vi "Protocol.Main.vi"(10 "Parameters":variant, 11 "Process":refnum<class "Process.lvclass">) -> ()   [LabVIEW 2023, in "J1939 Addon Engine.lvlib"]
uses:
  J1939 Addon Engine.lvlib
  <vilib>/NI/NIVS Inline Async API/_VS Inline Async API/Process/Process.lvclass
  Types/Protocol.App Settings.ctl
  Addon Shared/Types/XNET Settings.ctl
  Addon Shared/Types/Monitor Settings.ctl
  Types/Protocol.XNET Refs.ctl
  <vilib>/NI VeriStand/Custom Device API/Block Data Reference.ctl
  <vilib>/NI VeriStand/Custom Device API/Data Reference.ctl
  Types/Main.Outgoing.Frame.Settings.ctl
  Addon Shared/Types/Outgoing Event Trigger Types.ctl
  SubModules/Frame-Protection-Support/Source/Shared/Types/Exported Frame Settings.ctl
  SubModules/Frame-Protection-Support/Source/Shared/Types/Exported Frame Type.ctl
  SubModules/Frame-Protection-Support/Source/Shared/Types/Exported Protection Settings.ctl
  SubModules/Frame-Protection-Support/Source/Shared/Types/Protection Type.ctl
  SubModules/Frame-Protection-Support/Source/Shared/Types/XNET Signal Configuration.ctl
  SubModules/Frame-Protection-Support/Source/Shared/Types/Exported Counter Settings.ctl
  SubModules/Frame-Protection-Support/Source/Shared/Types/Exported Event Trigger Type.ctl
  Types/Engine.DTC Settings.ctl
  Addon Shared/Types/Compiled Simulated Settings.ctl
  Types/Engine.DTC FIFOs.ctl
  <vilib>/NI/NIVS Inline Async API/_VS Inline Async API/Process/Process.lvclass/Process.ctl
  <vilib>/NI/NI VeriStand Addon Network Comm/Engine/VeriStand Comm.lvclass/VeriStand Comm.ctl
  SubVIs/Protocol.Process Incoming Messages.vi
  <vilib>/NI/NIVS Inline Async API/_VS Inline Async API/Process/Methods/Async.Processes.Report.vi
  <vilib>/NI/NI VeriStand Addon Network Comm/Engine/_SubVIs/Comm Connection Engine.vi
  <vilib>/NI/NI VeriStand Addon Network Comm/Engine/_SubVIs/Comm Command Engine.vi
  SubVIs/Protocol.Process J1939 Incoming Messages.vi
  SubVIs/Protocol.RQST Lookup Table Act.vi
  <vilib>/NI/NI VeriStand Addon Network Comm/Engine/Comm API/Read Command.vi
  SubVIs/Protocol.RQST Wait on Response.vi
  SubVIs/Protocol.RQST Wait on Multiple Requests.vi
  Support Libraries/J1939 Utilities/Common Conversions.vi
  Support Libraries/J1939 Utilities/SubVIs/Convert CAN Arb ID to J1939 ID.vi
  SubModules/CAN-Streaming-Support/Source/Addon/Addon Engine/SubVIs/Reset Engine Stream Filter.vi
  SubModules/CAN-Streaming-Support/Source/Addon/Addon Engine/SubVIs/Get Engine Stream Filter.vi
  SubModules/CAN-Streaming-Support/Source/Addon/Addon Engine/SubVIs/Set Engine Stream Filter.vi
  SubVIs/Format Debug String.vi
  SubVIs/Protocol.Address Lookup Table Action.vi
  <vilib>/NI/NI VeriStand Addon Network Comm/Engine/Comm API/Respond to Command.vi
  <vilib>/Utility/error.llb/Clear Errors.vi
  SubModules/CAN-Streaming-Support/Source/Addon/Addon Engine/SubVIs/Engine Steam Format Debug String.vi
  SubModules/CAN-Streaming-Support/Source/Addon/Addon Engine/SubVIs/CAN Frame Filter.vi
  SubVIs/Protocol.Filter by Device Address.vi
  SubVIs/Protocol.Process Incoming Messages by PDU F.vi
  <vilib>/NI/NIVS Inline Async API/_VS Inline Async API/Error Handling Process/SubVIs/Error.ConvertArray.vi
  <vilib>/NI/STM/Connection Manager/TCP/Advanced/TCP Connection Manager (By Reference).vi
  <vilib>/NI/STM/Get Connection Reference.vi
  <vilib>/NI/STM/TCP/Get Connection Reference (TCP).vi
  <vilib>/NI/STM/Read Meta Data.vi
  <vilib>/NI/STM/TCP/Read Meta Data (TCP Ref).vi
  <vilib>/NI/AMC/Send Local Message.vi
  <vilib>/NI/Tools/Keyed Array/Add.vi
  <vilib>/NI/AMC/Read Next Message.vi
  <vilib>/NI/STM/Connection Manager/TCP/Advanced/TCP Check Connection (By Reference).vi
  SubVIs/Protocol.J1939 Filter by Device Address.vi
  <vilib>/NI/Tools/Keyed Array/Index.vi
  Support Libraries/J1939 Utilities/Common Messages.vi
  Support Libraries/J1939 Utilities/SubVIs/Request.vi
  SubVIs/Protocol.Parse Message Type.vi
  SubVIs/Protocol.RQST Look for Response.vi
  Support Libraries/J1939 Utilities/SubVIs/Convert J1939 ID to CAN Arb ID.vi
  Support Libraries/J1939 Utilities/SubVIs/Convert CAN Data (U32) to U8.vi
  SubVIs/Protocol.Get Simulated Previously Active DTCs.vi
  SubVIs/Protocol.Get Simulated Active DTCs.vi
  Support Libraries/J1939 Utilities/SubVIs/Acknowledgement.vi
  SubVIs/Protocol.Send Reset Previously Active DTC to Main.vi
  SubVIs/Protocol.Send Reset Active DTC to Main.vi
  SubVIs/Protocol.Convert Signals to Frame by ID.vi
  <vilib>/NI/STM/SubVIs/Generate STM Error.vi
  <vilib>/NI/AMC/Create Single Message.vi
  <vilib>/NI/AMC/Update Message Routing Info.vi
  <vilib>/NI/Tools/Keyed Array/Map String.vi
  <vilib>/NI/AMC/Read Termination Message.vi
  SubVIs/Protocol.Convert Data to DTC Frame.vi
  <vilib>/NI/Tools/String/Get Case Matching.vi
  <vilib>/xnet/xnet.llb/XNET Create Session.vi
  <vilib>/xnet/xnet.llb/XNET Create Session (Frame Input Stream).vi
  <vilib>/Utility/SystemLogging/Write to System Log.vi
  <vilib>/xnet/xnet.llb/XNET Read.vi
  <vilib>/xnet/xnet.llb/XNET Read (Frame CAN).vi
  <vilib>/xnet/xnet.llb/XNET Read (State CAN Comm).vi
  <vilib>/xnet/xnet.llb/XNET Clear.vi
  <vilib>/NI/NI VeriStand Addon Network Comm/Shared/Comm Constants.vi
  <vilib>/NI/AMC/Globals.vi
  <vilib>/Utility/error.llb/Error Cluster From Error Code.vi
  SubVIs/Protocol.RQST Lookup Table.vi
  SubVIs/Protocol.Address Lookup Table.vi
  <vilib>/NI/AMC/Send Message.vi
  <vilib>/xnet/xnet.llb/XNET Create Session (Conversion).vi
  <vilib>/xnet/xnet.llb/XNET Convert.vi
  <vilib>/xnet/xnet.llb/XNET Convert (Signal to Frame CAN).vi
  <vilib>/NI/STM/Read Message.vi
  <vilib>/NI/STM/TCP/Read Message (TCP).vi
  <vilib>/NI/AMC/Create Message Queue.vi
  <vilib>/NI/STM/Write Message.vi
  <vilib>/NI/STM/TCP/Write Message (TCP).vi
  <vilib>/NI/AMC/Destroy Message Queue.vi
  <vilib>/NI/STM/TCP/Read Meta Data (TCP Clst).vi
  SubVIs/Protocol.Close References.vi
  <vilib>/NI/NI VeriStand Addon Network Comm/Engine/Process/Close Comm Refs.vi
  <vilib>/NI/NI VeriStand Addon Network Comm/Engine/VeriStand Comm.lvclass
  Addon Shared/J1939 Addon Shared.lvlib
  <vilib>/NI VeriStand/Custom Device API/Custom Device API.lvlib
  SubModules/Frame-Protection-Support/Source/Shared/Protection and Counter Support Shared.lvlib
  SubModules/CAN-Streaming-Support/Source/Addon/Addon Engine/CAN Stream Support Engine.lvlib
panel:
  out "error out":errorcluster
  # "CONTROL & MONITORING"
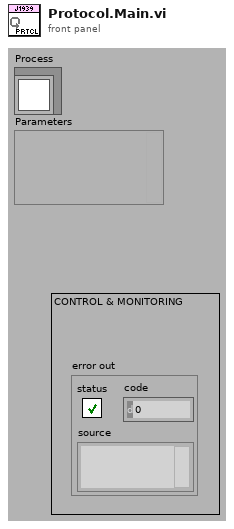
[diagram p1: front panel]
types:
  T1 = typedef "J1939 Addon Engine.lvlib/Protocol.App Settings.ctl" = cluster{"Name":string, "XNET.Settings":T2, "Monitor.Network":T3, "Data":T4[], "DTCs":T16[], "Sim.Nodes.LUT":variant, "Data.LUT":variant, "PCL":u32}
  T2 = typedef "J1939 Addon Shared.lvlib/XNET Settings.ctl" = cluster{"Database":refnum<k21>, "Cluster":refnum<k21>, "Port":string, "Baud rate [Bd]":u32, "Termination":u32, "Incoming Decimation":u32, "Outgoing Decimation":u32}
  T3 = typedef "J1939 Addon Shared.lvlib/Monitor Settings.ctl" = cluster{"Address":u8, "Name":u64, "Include DA":bool, "Force SA":bool}
  T4 = typedef "J1939 Addon Engine.lvlib/Protocol.XNET Refs.ctl" = cluster{"Network":T3, "Incoming.Use":bool, "Incoming.Session":refnum<k21>, "Incoming.Refs":T5[], "Incoming.Values":dbl[], "Outgoing.Frames":T7[], "Outgoing.Initialize":bool, "Outgoing.Refs":T5[], "Outgoing.Values":dbl[], "Request.Table":refnum<k33>, "Timing.Use":bool, "Timing.Index":i32[], "Timing.Refs":T5[], "Timing.Values":dbl[], "Disable.Refs":T5[], "Disable.Values":dbl[], "Trigger.Refs":T5[], "Trigger.Values":dbl[], "Outgoing.Frames.CountersAndProtections":T9[]}
  T5 = typedef "Custom Device API.lvlib/Block Data Reference.ctl" = cluster{"Data Reference":T6, "Offset":u64, "Length":u64}
  T6 = typedef "Custom Device API.lvlib/Data Reference.ctl" = i32
  T7 = typedef "J1939 Addon Engine.lvlib/Main.Outgoing.Frame.Settings.ctl" = cluster{"Offset":u32, "Length":u32, "Cyclic":bool, "Disable.Index":i32, "Disable":bool, "Trigger":T8, "Trigger.Index":i32, "Session":refnum<k21>}
  T8 = typedef "J1939 Addon Shared.lvlib/Outgoing Event Trigger Types.ctl" = enum16{"Channel value change", "Trigger channel (not zero)", "Channel value change or trigger channel (not zero)", "Trigger channel (any value change)", "Channel value change or trigger channel (any value change)"}
  T9 = typedef "Protection and Counter Support Shared.lvlib/Exported Frame Settings.ctl" = cluster{"Type":T10, "Frame ID":u32, "Payload Length":u32, "Signal XNET Paths":string[], "Frame.PrevData":dbl[], "VS Offset":i32, "VS Length":i32, "Generation Period":u32, "Has Protection?":bool, "Protection Configurations":T11[], "Has Counter":bool, "Counter Configurations":T14[], "Has Disable?":bool, "Disable VS Index":i32, "Transmit Trigger":T15, "Trigger VS Index":i32}
  T10 = typedef "Protection and Counter Support Shared.lvlib/Exported Frame Type.ctl" = enum16{"Periodic", "Event", "Periodic/Event"}
  T11 = typedef "Protection and Counter Support Shared.lvlib/Exported Protection Settings.ctl" = cluster{"Protection Frame Index":i32, "Protection Type":T12, "Data Indeces":i32[], "Initialized Data Array":dbl[], "Protection Signal XNET Paths":string[], "CRC Channels":T13[], "Protection VS Update Index":i32, "Override Index":i32, "Override Value Index":i32}
  T12 = typedef "Protection and Counter Support Shared.lvlib/Protection Type.ctl" = enum16{"Arb ID + Bytes Checksum with Inversion", "Arb ID + Bytes CRC with Inversion", "Reversed Raw Signal Checksum with Inversion", "Concatenated Two's Compliment"}
  T13 = typedef "Protection and Counter Support Shared.lvlib/XNET Signal Configuration.ctl" = cluster{"Start Bit":i32, "Name":string, "Number of bits":i32, "Scale":dbl, "Offset":dbl, "Data Type":u32, "Counter":bool}
  T14 = typedef "Protection and Counter Support Shared.lvlib/Exported Counter Settings.ctl" = cluster{"Frame Index":i32, "Max Count":dbl, "VS Index":i32, "Bit Length":i64, "Override Index":i32, "Override Value Index":i32}
  T15 = typedef "Protection and Counter Support Shared.lvlib/Exported Event Trigger Type.ctl" = enum16{"Channel value change", "Trigger channel (not zero)", "Channel value change or trigger channel (not zero)", "Trigger channel (any value change)", "Channel value change or trigger channel (any value change)"}
  T16 = typedef "J1939 Addon Engine.lvlib/Engine.DTC Settings.ctl" = cluster{"Data":T17, "FIFOs":T18}
  T17 = typedef "J1939 Addon Shared.lvlib/Compiled Simulated Settings.ctl" = cluster{"DM1.Ref":T5[], "DM1.Value":dbl[], "DM1.Enable.Ref":T5[], "DM1.Enable.Value":dbl[], "DM2.Ref":T5[], "DM2.Value":dbl[], "DM2.Enable.Ref":T5[], "DM2.Enable.Value":dbl[]}
  T18 = typedef "J1939 Addon Engine.lvlib/Engine.DTC FIFOs.ctl" = cluster{"DM1.Data":refnum<k33>, "DM1.Enable":refnum<k33>, "DM2.Data":refnum<k33>, "DM2.Enable":refnum<k33>, "DM1.Reset":refnum<k33>, "DM2.Reset":refnum<k33>}
  T19 = typedef "J1939 Addon Engine.lvlib/Protocol.Configuration.ctl" = cluster{"Refs":T20, "XNET":T23, "Comm":refnum<class "VeriStand Comm.lvclass">, "Process":refnum<class "Process.lvclass">, "Name":string, "InternalCmd":T24, "InternalResp":T25, "Resp.Data":dbl[], "CounterProtection":T26[], "Stream Refs":T29}
  T20 = typedef "J1939 Addon Engine.lvlib/Protocol.Refs.ctl" = cluster{"Processed Outgoing":refnum<queue>, "Simulated Addresses LUT":variant, "Data LUT":variant, "RequestDataTables":refnum<k33>[], "RQST":T21, "Address LUT":T22, "Addresses":u8[], "Monitor Address":u8}
  T21 = typedef "J1939 Addon Engine.lvlib/Protocol.RQST Lookup Table Reference.ctl" = refnum<data-value>
  T22 = typedef "J1939 Addon Engine.lvlib/Protocol.Address Table Reference.ctl" = refnum<data-value>
  T23 = typedef "J1939 Addon Engine.lvlib/Protocol.XNET Settings.ctl" = cluster{"Raw CAN In":refnum<k21>, "Raw Frames out":refnum<k21>[], "Raw J1939 In":refnum<k21>}
  T24 = typedef "Data Access Engine.lvlib/Data Access Engine.lvclass/Read.DVR.ctl" = refnum<data-value>
  T25 = typedef "Data Access Engine.lvlib/Data Access Engine.lvclass/Write.DVR.ctl" = refnum<data-value>
  T26 = typedef "J1939 Addon Engine.lvlib/CounterAndProtectionFrames.ctl" = cluster{"Frame Count":i32, "Frames in":T27[], "Protections":T25, "Signals":T24, "Overrides":T24}
  T27 = typedef "Protection and Counter Support Engine.lvlib/RT Frame Settings.ctl" = cluster{"Type":T10, "Frame ID":u32, "Payload Length":u32, "VS Offset":i32, "VS Length":i32, "Frame Conversion":refnum<k21>, "Frame.Data":dbl[], "Generation Period":u32, "Time Since Last Generation":u32, "Generation Iterations":u32, "Generation Counter":u32, "Has Protection?":bool, "Protection Configurations":T28[], "Has Counter?":bool, "Counter Configurations":T14[], "Has Disable?":bool, "Disable VS Index":i32, "Transmit Trigger":T15, "Trigger VS Index":i32}
  T28 = typedef "Protection and Counter Support Engine.lvlib/RT Protection Configuration.ctl" = cluster{"Protection Frame Index":i32, "Protection Type":T12, "Data Indeces":i32[], "Data Array":dbl[], "Check Sum Conversion":refnum<k21>, "CRC Channels":T13[], "Protection VS Index":i32, "Counter Data Index":i32, "Override Index":i32, "Override Value Index":i32}
  T29 = typedef "CAN Stream Support Engine.lvlib/Engine Stream Refs.ctl" = cluster{"Addon":string, "Port":refnum<k21>, "Filter Ref":refnum<data-value>, "Default Filter":T30, "Port Settings":T33}
  T30 = typedef "CAN Stream Support Shared.lvlib/Filter Parameters.ctl" = cluster{"ID Filters":u32[], "Direction Filter":T31, "Type Filter":T32}
  T31 = typedef "CAN Stream Support Shared.lvlib/Direction Filter.ctl" = enum16{"Tx/Rx", "Rx", "Tx"}
  T32 = typedef "CAN Stream Support Shared.lvlib/Type Filter.ctl" = enum16{"All", "CAN Data", "CAN Remote", "CAN Bus Error", "CAN 2.0 Data", "CAN FD Data", "CAN FD+BRS Data", "J1939 Data", "Delay", "Log Trigger", "Start Trigger"}
  T33 = typedef "CAN Stream Support Engine.lvlib/Engine Stream Port Settings.ctl" = cluster{"Mode":u32, "Baud Rate":u64, "Termination":u32, "FD ISO Mode":u32, "FD Baud Rate":u64}
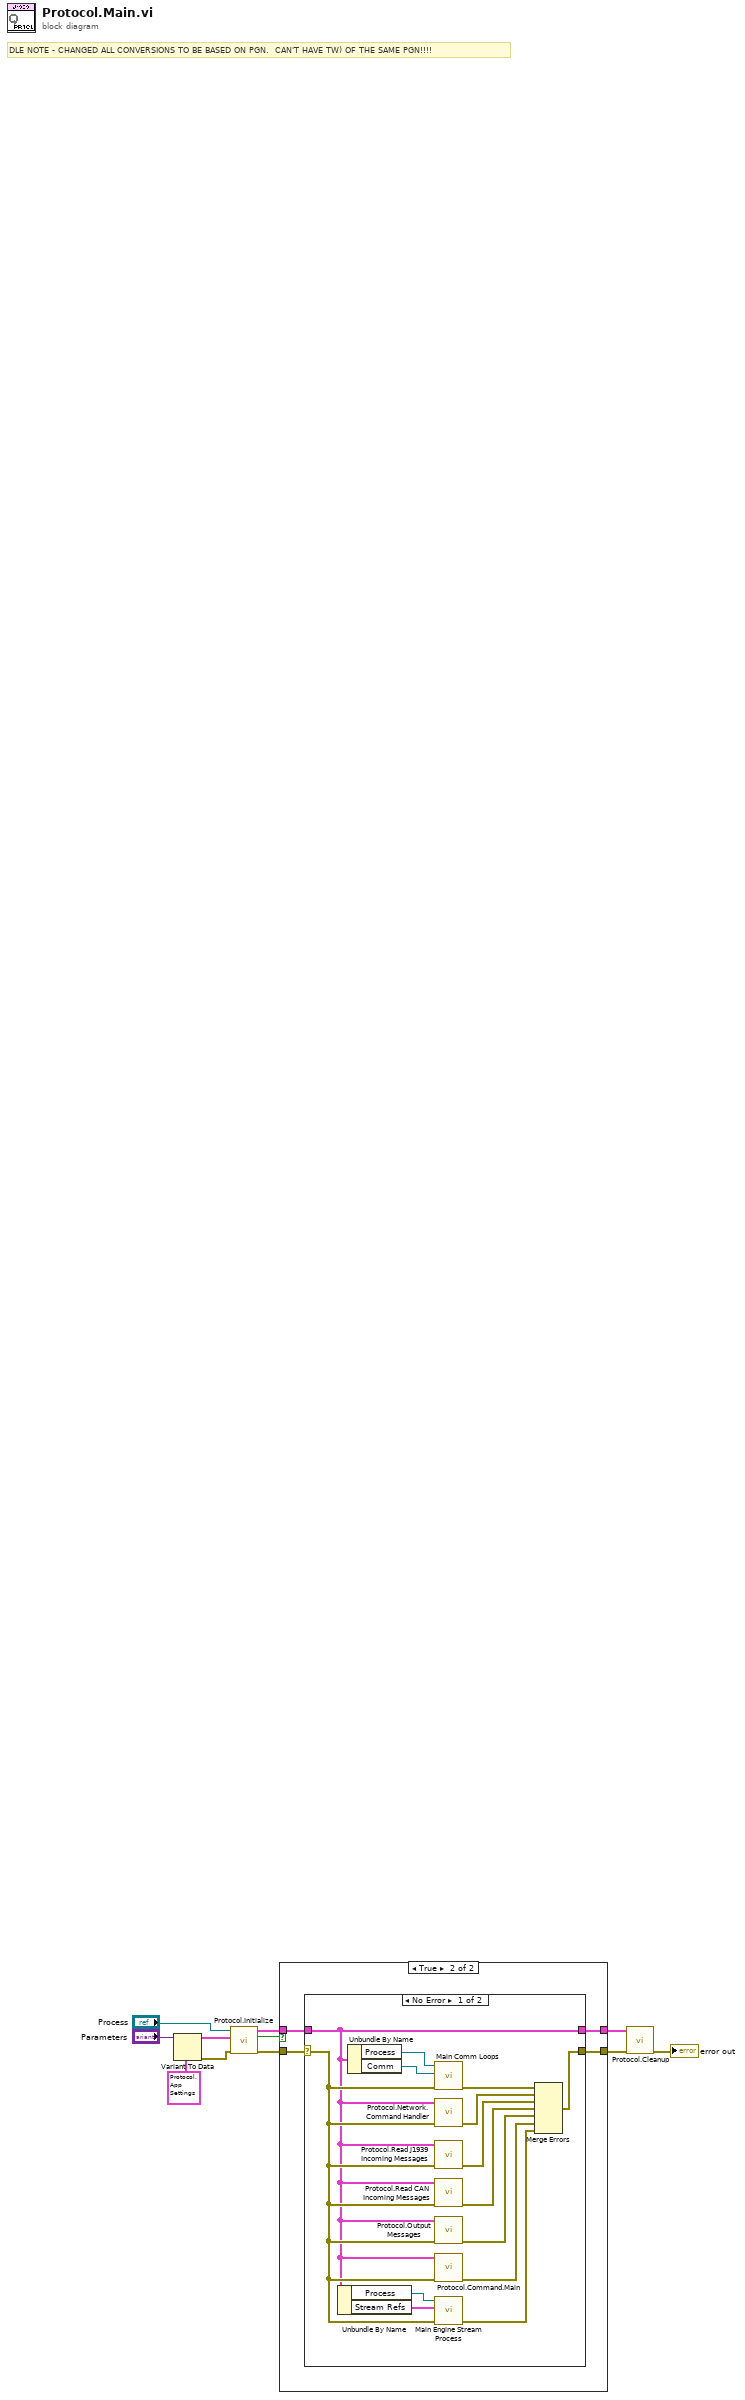
[diagram p0: block diagram]
diagram:
  # "DLE NOTE - CHANGED ALL CONVERSIONS TO BE BASED ON PGN.  CAN'T HAVE TW) OF THE SAME PGN!!!!"
  n1 = Variant To Data(type=T1 {"Name"="", "XNET.Settings"={"Database"="", "Cluster"="", "Port"="", "Baud rate [Bd]"=0, "Termination"=0, "Incoming Decimation"=0, "Outgoing Decimation"=1}, "Monitor.Network"={"Address"=0, "Name"=0, "Include DA"=FALSE, "Force SA"=FALSE}, "Data"=[], "DTCs"=[], "Sim.Nodes.LUT"=variant, "Data.LUT"=variant, "PCL"=0} ("Parameters"), Variant="Parameters") -> (data=w1:T1, error out=w2:errorcluster)  [unwired: 1 in]
  n2 = call "Protocol.Initialize.vi"("error in (no error)"=w2, "Parameters in"=w1, "Process"="Process") -> ("error out"=w11:errorcluster, "Notification"=w8:bool, "Protocol State Variables"=w7:T19)  [unwired: 6 in]
  n3 = case shown="True" w8 {
    tunnel: w11 -> [w13 w14]
    tunnel: [w13 w17] -> w10
    tunnel: w7 -> [w12 w15]
    tunnel: [w12 w16] -> w6
    frame False {
    }
    frame True {
      n4 = case shown="No Error" w14 {
        selector: w14 -> [w22 w33]
        tunnel: [w31 w33] -> w17
        tunnel: w15 -> [w21 w32]
        tunnel: [w21 w32] -> w16
        frame No Error {
          n5 = Unbundle By Name(w21) -> ("Process"=w20:refnum<class "Process.lvclass">, "Stream Refs"=w19:T29)
          n6 = Unbundle By Name(w21) -> ("Process"=w27:refnum<class "Process.lvclass">, "Comm"=w28:refnum<class "VeriStand Comm.lvclass">)
          n7 = call <vilib>:"Main Comm Loops.vi"("error in (no error)"=w22, "Comm.lvclass"=w28, "Process"=w27) -> ("error out"=w25:errorcluster)  [unwired: 8 in]
          n8 = call "Protocol.Network.Command Handler.vi"("error in (no error)"=w22, "J1939 Main Configuration"=w21) -> ("error out"=w26:errorcluster)  [unwired: 9 in]
          n9 = call "Protocol.Read J1939 Incoming Messages.vi"("error in (no error)"=w22, "J1939 Main Configuration"=w21) -> ("error out"=w24:errorcluster)  [unwired: 9 in]
          n10 = call "Protocol.Read CAN Incoming Messages.vi"("error in (no error)"=w22, "J1939 Main Configuration"=w21) -> ("error out"=w30:errorcluster)  [unwired: 9 in]
          n11 = call "Protocol.Output Messages.vi"("error in (no error)"=w22, "J1939 Main Configuration"=w21) -> ("error out"=w29:errorcluster)  [unwired: 9 in]
          n12 = call "Protocol.Command.Main.vi"("Error"=w22, "J1939 Main Configuration"=w21) -> ("error out"=w23:errorcluster)  [unwired: 9 in]
          n13 = call "Main Engine Stream Process.vi"("error in (no error)"=w22, "Refs"=w19, "Process in"=w20) -> ("error out"=w18:errorcluster)  [unwired: 8 in]
          n14 = Merge Errors(w25, w26, w24, w30, w29, w23, w18) -> (w31:errorcluster)
        }
        frame Error {
        }
      }
    }
  }
  n15 = call "Protocol.Cleanup.vi"("error in (no error)"=w10, "J1939 Main Configuration"=w6) -> ("error out"=→"error out":errorcluster)  [unwired: 9 in]
